vi "Main Remote Panel UI.vi"() -> ()   [LabVIEW 2019]
uses:
  Support/Main Loop States.ctl
panel:
  in  "VI Name":T1(ring)
  in  "Connect":bool
  in  "Server Port":i32=8000
  in  "Server Address":string="10.101.127.208"
  # "Client App Run on PC"
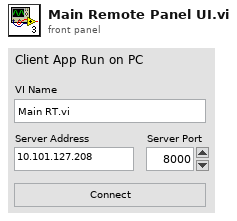
[diagram p1: front panel]
types:
  T1 = enum16{"Main RT.vi", "Example SubVI.vi", "Caveat 1.vi", "Caveat 1 Fix.vi", "Caveat 2.vi", "Caveat 2 Fix.vi"}
  T2 = typedef "Main Loop States.ctl" = enum16{"Idle", "Init", "Connect", "Error", "Exit"}
  T3 = enum32{"invalid app kind", "Development System", "Run Time System", "Student Edition", "Embedded LabVIEW", "Evaluation", "Custom"}
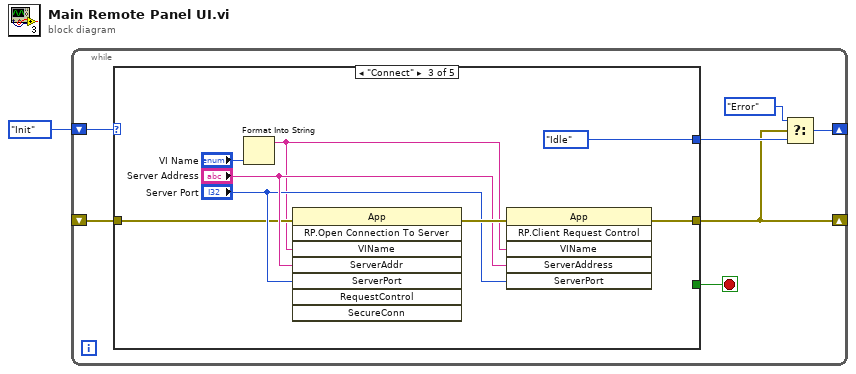
[diagram p0: block diagram]
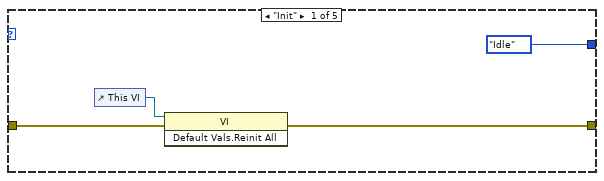
[diagram p2: hidden frame]
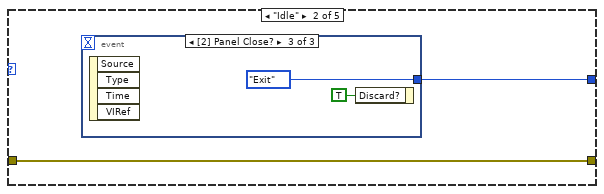
[diagram p3: hidden frame]
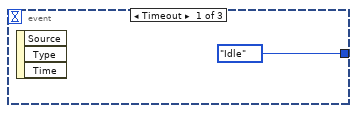
[diagram p4: hidden frame]
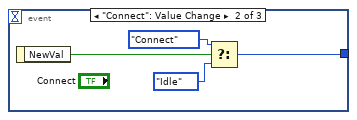
[diagram p5: hidden frame]
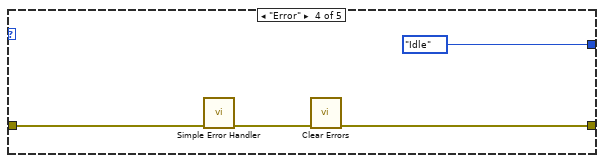
[diagram p6: hidden frame]
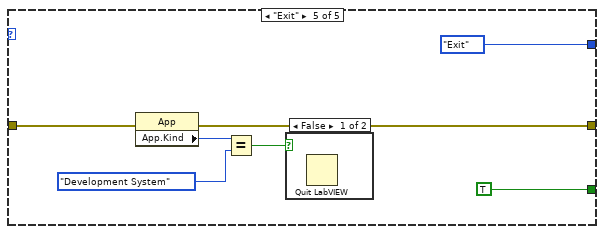
[diagram p7: hidden frame]
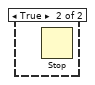
[diagram p8: hidden frame]
diagram:
  n1 = while {
    shift-right: [w5] -> _
    shift-left: Main_Loop_States."Init" -> [w8]
    shift-right: [w4] -> _
    shift-left: _ -> [w3]
    stop <- w2 stop-if-true
    n2 = case shown="\"Connect\"" w8 {
      tunnel: [w11 w13 w25 w31 w36] -> w4
      tunnel: [Main_Loop_States."Idle" ("f") w14 Main_Loop_States."Idle" Main_Loop_States."Idle" Main_Loop_States."Exit"] -> w6
      tunnel: w3 -> [w9 w13 w24 w33 w37]
      tunnel: [_ _ _ _ TRUE ("Stop")] -> w2
      frame "Init" {
        n3 = control-ref of="This VI"() -> (w12:refnum<vi>)
        n4 = invoke class="VI" method="Default Vals.Reinit All"(reference=w12, error in=w9) -> (error out=w11:errorcluster)  [unwired: 1 in, 2 out]
      }
      frame "Idle" {
        n5 = event shown="[2] Panel Close?" {
          selector: _ -> [_ _ _]
          dyn-events: _ -> [_ _ _]
          timeout: _ -> [_ _ _]
          tunnel: [Main_Loop_States."Idle" w17 Main_Loop_States."Exit"] -> w14
          event Timeout {
            n6 = event-data() -> ()  [unwired: 1 in, 3 out]
          }
          event "Connect": Value Change {
            n7 = event-data() -> ("NewVal"=w18:bool)  [unwired: 1 in]
            n8 = Select(t=Main_Loop_States."Connect", s=w18, f=Main_Loop_States."Idle") -> (s? t:f=w17:T2)
          }
          event Panel Close? {
            n9 = event-data() -> ()  [unwired: 1 in, 4 out]
            n10 = event-data("Discard?"=TRUE) -> ()  [unwired: 1 in, 1 out]
          }
        }
      }
      frame "Connect" {
        n11 = Format Into String("VI Name") -> (resulting string=w22:string)  [unwired: 3 in, 1 out]
        n12 = invoke class="App" method="RP.Open Connection To Server"(error in=w24, "VIName"=w22, "ServerAddr"="Server Address", "ServerPort"="Server Port") -> (error out=w28:errorcluster)  [unwired: 4 in, 7 out]
        n13 = invoke class="App" method="RP.Client Request Control"(error in=w28, "VIName"=w22, "ServerAddress"="Server Address", "ServerPort"="Server Port") -> (error out=w25:errorcluster)  [unwired: 2 in, 5 out]
      }
      frame "Error" {
        n14 = call <vilib>:"Simple Error Handler.vi"("error in (no error)"=w33) -> ("error out"=w32:errorcluster)  [unwired: 4 in, 4 out]
        n15 = call <vilib>:"Clear Errors.vi"("error in (no error)"=w32) -> ("error out"=w31:errorcluster)  [unwired: 5 in, 1 out]
      }
      frame "Exit" {
        n16 = property class="App"(error in=w37) -> (error out=w36:errorcluster, "App.Kind"=w40:T3)  [unwired: 1 in, 1 out]
        n17 = Equal?(x=w40, y=T3."Development System" ("Application:Kind")) -> (x = y?=w38:bool)
        n18 = case shown="False" w38 {
          frame False {
            n19 = Quit LabVIEW() -> ()  [unwired: 1 in]
          }
          frame True {
            n20 = Stop() -> ()  [unwired: 1 in]
          }
        }
      }
    }
    n21 = Select(t=Main_Loop_States."Error", s=w4, f=w6) -> (s? t:f=w5:T2)
  }
